vi "EtalonnageStub.vi"(6 "XY Graph":refnum<vi>, 7 "Reference Cell":i32=1, 8 "error in":errorcluster, 9 "Volume":dbl format="%#_13g", 10 "Over":bool=TRUE, 11 "NextStep":bool=TRUE) -> (0 "error out":errorcluster, 1 "Résidu":dbl, 2 "CoeffsPoly":dbl[](array[numeric]), 3 "Values":cluster{dbl[], dbl[]})   [LabVIEW 2013]
uses:
  MeasureStateStub.vi
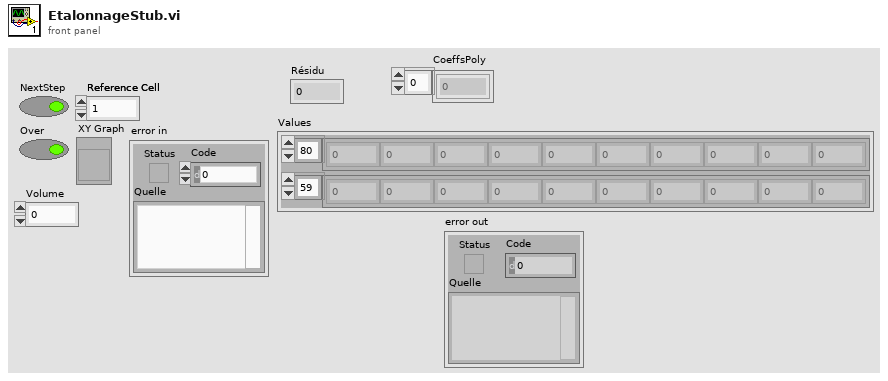
[diagram p1: front panel]
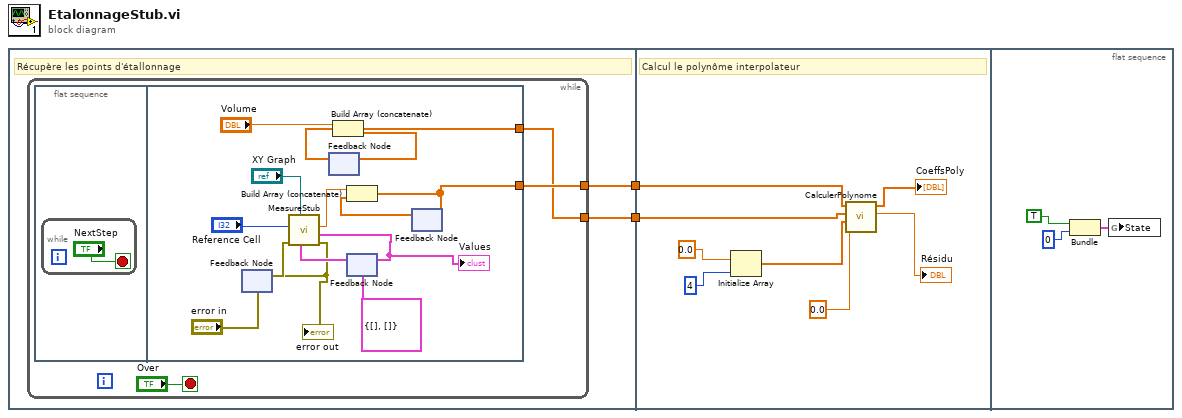
[diagram p0: block diagram]
diagram:
  n1 = flat-sequence {
    tunnel: [w4] -> w2
    tunnel: [w3] -> w1
    tunnel: w2 -> [w24]
    tunnel: w1 -> [w23]
    frame #0 {
      # "Récupère les points d'étallonnage"
      n2 = while {
        tunnel: [w7] -> w4
        tunnel: [w5] -> w3
        stop <- "Over" stop-if-true
        n3 = flat-sequence {
          tunnel: [w16] -> w7
          tunnel: [w9] -> w5
          frame #0 {
            n4 = while {
              stop <- "NextStep" stop-if-true
            }
          }
          frame #1 {
            n5 = feedback #1("error in") -> (w22:errorcluster)
            n6 = feedback #2() -> (w18:dbl[])  [unwired: 1 in]
            n7 = Build Array (concatenate)("Volume", w18) -> (w9:dbl[])
            n8 = feedback-in #2(w9) -> ()
            n9 = feedback #3(cluster{dbl[], dbl[]} {[], []}) -> (w21:cluster{dbl[], dbl[]})
            n10 = call "MeasureStub.vi"("Graph in"=w21, "XY Graph"="XY Graph", "error in"=w22, "Reference Cell"="Reference Cell") -> ("error out"=w10:errorcluster, "Values"=w11:cluster{dbl[], dbl[]}, "P1/P2"=w20:dbl)  [unwired: 5 in]
            "Values" <- w11
            "error out" <- w10
            n11 = feedback-in #1(w10) -> ()
            n12 = feedback-in #3(w11) -> ()
            n13 = feedback #4() -> (w19:dbl[])  [unwired: 1 in]
            n14 = Build Array (concatenate)(w20, w19) -> (w16:dbl[])
            n15 = feedback-in #4(w16) -> ()
          }
        }
      }
    }
    frame #1 {
      # "Calcul le polynôme interpolateur"
      n16 = Initialize Array(0.0, 4) -> (w28:dbl[])
      n17 = call "CalculerPolynome.vi"("e3 [in]"=0.0, "Meilleure poly [in]"=w28, "Y"=w23, "X"=w24) -> ("Résidu [out]"=→"Résidu":dbl, "Meilleur poly [out]"=→"CoeffsPoly":dbl[])  [unwired: 6 in]
    }
    frame #2 {
      n18 = Bundle(TRUE, 0) -> (w33:cluster{bool, i32})  [unwired: 1 in]
      n19 = global write "MeasureStateStub.vi" "State"(w33) -> ()
    }
  }
